vi "Measurement Logic.vi"(8 "error in":errorcluster, 10 "Measurement Context":refnum<class "MeasurementContext.lvclass">, 11 "Measurement Configuration":T2={"delay"=10.0}) -> (0 "error out":errorcluster, 2 "Measurement Context out":refnum<class "MeasurementContext.lvclass">, 3 "Measurement Results":T1)   [LabVIEW 2020, in "CancellableMeasurementProxy.lvlib"]
uses:
  CancellableMeasurementProxy.lvlib
  Measurement Configuration.ctl
  Measurement Results.ctl
  RPC Service/MeasurementContext/MeasurementContext.lvclass
  <vilib>/MeasurementLink/Discovery Client/RPC Messages/ni_measurementlink_discovery_v1_ResolveServiceRequest.ctl
  Measurement Client_lv/Measurement_client/RPC Messages/ni_measurementlink_measurement_v1_MeasureRequest.ctl
  Measurement Client_lv/Measurement_client/RPC Messages/google_protobuf_Any.ctl
  Measurement Client_lv/Measurement_client/RPC Messages/ni_measurementlink_PinMapContext.ctl
  5cd0f8b4-e5f8-4204-8add-725bbbd3d453.vi
  d93fa0da-b198-4c2c-a1c3-c340aeb95d8d.vi
  <vilib>/gRPC/LabVIEW gRPC Library/Server API/Translate Protobuf Error.vi
  <vilib>/AdvancedString/1D String Array to Delimited String.vi
  <vilib>/gRPC/LabVIEW gRPC Library/Server API/Server/Get Server DLL Path.vi
  RPC Service/MeasurementContext/Accessor/Is Canceled.vi
  <vilib>/MeasurementLink/Discovery Client/Discovery_client.lvlib
  Measurement Client_lv/Measurement_client/Measurement_client.lvlib
  <vilib>/gRPC/LabVIEW gRPC Library/grpc-lvsupport-release.lvlib
panel:
  out "target address":string
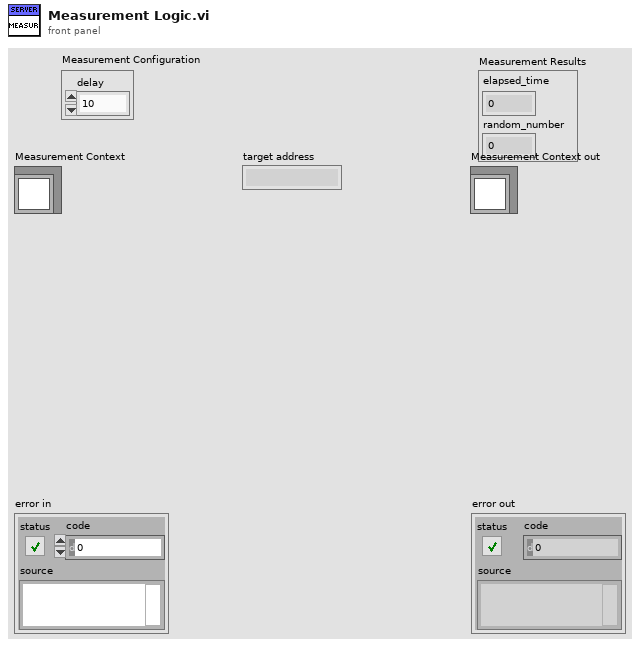
[diagram p1: front panel]
types:
  T1 = typedef "CancellableMeasurementProxy.lvlib/Measurement Results.ctl" = cluster{"elapsed_time":dbl, "random_number":dbl}
  T2 = typedef "CancellableMeasurementProxy.lvlib/Measurement Configuration.ctl" = cluster{"delay":dbl}
  T3 = typedef "Measurement_client.lvlib/ni_measurementlink_measurement_v1_MeasureRequest.ctl" = cluster{"configuration_parameters":T4, "pin_map_context":T5}
  T4 = typedef "Measurement_client.lvlib/google_protobuf_Any.ctl" = cluster{"type_url":string, "value":u8[]}
  T5 = typedef "Measurement_client.lvlib/ni_measurementlink_PinMapContext.ctl" = cluster{"pin_map_id":string, "sites":i32[]}
  T6 = typedef "Discovery_client.lvlib/ni_measurementlink_discovery_v1_ResolveServiceRequest.ctl" = cluster{"provided_interface":string, "service_class":string}
  T7 = typedef "grpc-lvsupport-release.lvlib/grpcId.ctl" = u64
  T8 = typedef "Discovery_client.lvlib/ni_measurementlink_discovery_v1_ServiceLocation.ctl" = cluster{"location":string, "insecure_port":string, "ssl_authenticated_port":string}
  T9 = typedef "grpc-lvsupport-release.lvlib/Any.ctl" = cluster{"Type Url":string, "Bytes":u8[]}
  T10 = typedef "Measurement_client.lvlib/ni_measurementlink_measurement_v1_MeasureResponse.ctl" = cluster{"outputs":T4}
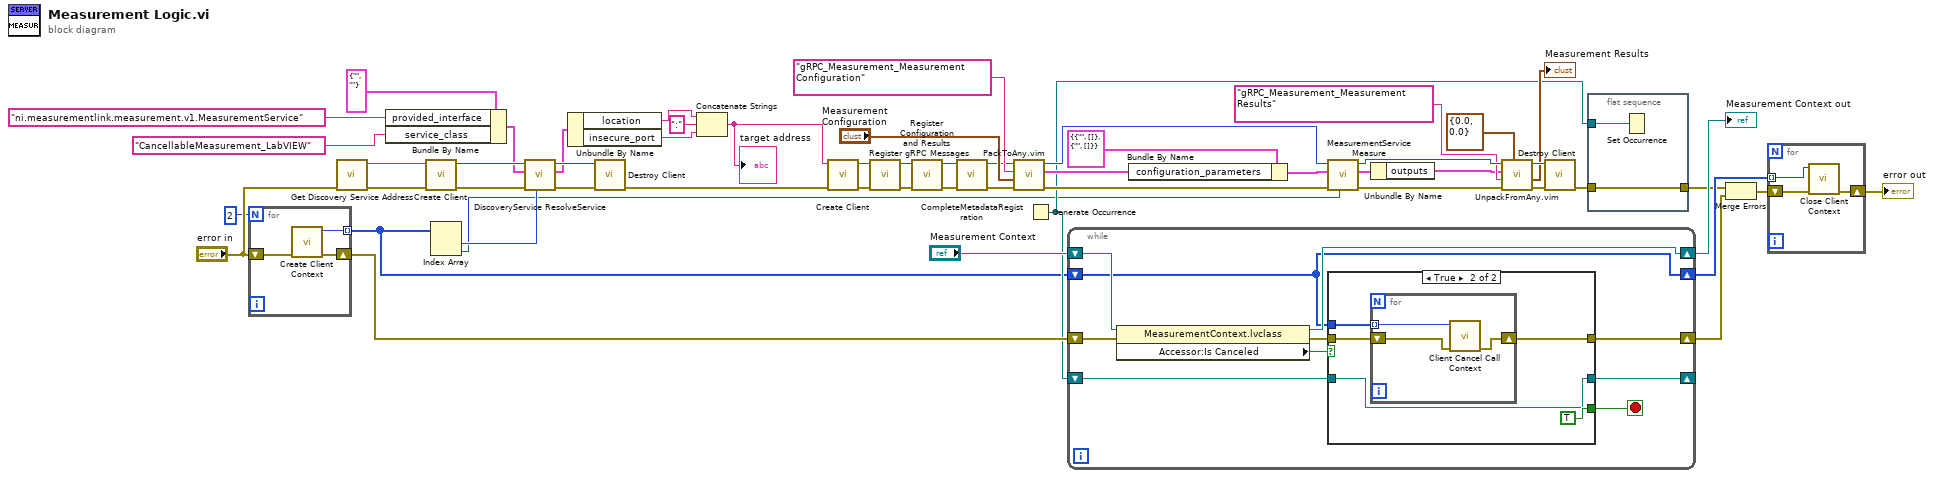
[diagram p0: block diagram]
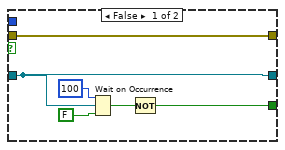
[diagram p2: hidden frame]
diagram:
  n1 = for {
    N: 2 -> [_]
    tunnel: [w57] -> w2 mode=indexing
    shift-right: [w56] -> w14
    shift-left: "error in" -> [w58]
    n2 = call <vilib>:"Create Client Context.vi"("error in (no error)"=w58) -> ("error out"=w56:errorcluster, "ContextID out"=w57:T7)  [unwired: 9 in]
  }
  n3 = call "Get Discovery Service Address.vi"("error in"="error in") -> ("error out"=w46:errorcluster, "address"=w55:string)  [unwired: 9 in]
  n4 = Bundle By Name(cluster=T6 {"provided_interface"="", "service_class"=""} ("Request Data"), "provided_interface"="ni.measurementlink.measurement.v1.MeasurementService", "service_class"="CancellableMeasurement_LabVIEW") -> (w52:T6)
  n5 = call <vilib>:"Create Client.vi"("error in"=w46, "address"=w55) -> ("error out"=w47:errorcluster, "gRPC ID Out"=w54:T7)  [unwired: 8 in]
  n6 = Index Array(array=w2) -> (element #1=w4:T7, element #2=w3:T7)  [unwired: 2 in]
  n7 = call <vilib>:"DiscoveryService ResolveService.vi"("contextId"=w4, "error in"=w47, "Request Data"=w52, "gRPC ID"=w54) -> ("error out"=w48:errorcluster, "Response Data"=w45:T8, "gRPC ID out"=w49:T7)  [unwired: 5 in]
  n8 = Unbundle By Name(w45) -> ("location"=w43:string, "insecure_port"=w42:string)
  n9 = call <vilib>:"Destroy Client.vi"("error in"=w48, "gRPC ID"=w49) -> ("error out"=w16:errorcluster)  [unwired: 9 in]
  n10 = Concatenate Strings(w43, ":" ("string"), w42) -> (w17:string)
  "target address" <- w17
  n11 = call <vilib>:"Create Client.vi"("error in"=w16, "address"=w17) -> ("error out"=w25:errorcluster, "ClientID out"=w24:T7)  [unwired: 8 in]
  n12 = call "Register gRPC Messages.vi"("error in (no error)"=w25, "gRPC ID"=w24) -> ("error out"=w22:errorcluster, "gRPC ID Out"=w23:T7)  [unwired: 8 in]
  n13 = call "Register Configuration and Results.vi"("error in (no error)"=w22, "gRPC ID"=w23) -> ("error out"=w21:errorcluster, "gRPC ID Out"=w20:T7)  [unwired: 8 in]
  n14 = call <vilib>:"CompleteMetadataRegistration.vi"("error in"=w21, "gRPC ID in"=w20) -> ("error out"=w18:errorcluster, "gRPC ID Out"=w19:T7)  [unwired: 8 in]
  n15 = call "PackToAny.vim"("error in"=w18, "Data To Pack"="Measurement Configuration", "Message Type"="gRPC_Measurement_Measurement Configuration", "gRPCid in"=w19) -> ("error out"=w28:errorcluster, "Any"=w36:T9, "gRPCid out"=w41:u64)  [unwired: 5 in]
  n16 = Generate Occurrence() -> (w9:refnum<k4>)
  n17 = while {
    shift-right: [w61] -> w13
    shift-left: w2 -> [w61]
    shift-right: [w65] -> w11
    shift-left: "Measurement Context" -> [w68]
    shift-right: [w63] -> w7
    shift-left: w14 -> [w66]
    shift-right: [w59] -> _
    shift-left: w9 -> [w60]
    stop <- w62 stop-if-true
    n18 = property class="MeasurementContext.lvclass"(reference=w68, error in=w66) -> (reference out=w65:refnum<class "MeasurementContext.lvclass">, error out=w64:errorcluster, "Accessor:Is Canceled"=w67:bool)
    n19 = case shown="True" w67 {
      tunnel: w61 -> [_ w79]
      tunnel: w64 -> [w74 w78]
      tunnel: [w74 w77] -> w63
      tunnel: [w71 TRUE] -> w62
      tunnel: w60 -> [w70 w75]
      tunnel: [w70 w75] -> w59
      frame False {
        n20 = Wait on Occurrence(1:FALSE ("ignore previous (T)"), 2:w70, 3:100 ("ms timeout (-1)")) -> (0:w72:bool)
        n21 = Not(x=w72) -> (.not. x?=w71:bool)
      }
      frame True {
        n22 = for {
          tunnel: w79 -> [w82] mode=indexing
          shift-right: [w80] -> w77
          shift-left: w78 -> [w81]
          n23 = call <vilib>:"Client Cancel Call Context.vi"("error in"=w81, "Call ID in"=w82) -> ("error out"=w80:errorcluster)  [unwired: 9 in]
        }
      }
    }
  }
  "Measurement Context out" <- w11
  n24 = Bundle By Name(cluster=T3 {"configuration_parameters"={"type_url"="", "value"=[]}, "pin_map_context"={"pin_map_id"="", "sites"=[]}} ("Request Data"), "configuration_parameters"=w36) -> (w37:T3)
  n25 = call "MeasurementService Measure.vi"("contextId"=w3, "error in"=w28, "Request Data"=w37, "gRPC ID"=w41) -> ("error out"=w27:errorcluster, "Response Data"=w33:T10, "gRPC ID out"=w35:T7)  [unwired: 5 in]
  n26 = Unbundle By Name(w33) -> ("outputs"=w32:T4)
  n27 = call "UnpackFromAny.vim"("Data Type"=T1 {"elapsed_time"=0.0, "random_number"=0.0} ("Measurement Results"), "error in"=w27, "Message Type"="gRPC_Measurement_Measurement Results", "Any"=w32, "gRPCid in"=w35) -> ("error out"=w26:errorcluster, "Unpacked Value"=→"Measurement Results":T1, "gRPCid out"=w31:u64)  [unwired: 4 in]
  n28 = call <vilib>:"Destroy Client.vi"("error in"=w26, "gRPC ID"=w31) -> ("error out"=w10:errorcluster)  [unwired: 9 in]
  n29 = flat-sequence {
    tunnel: [w84] -> w8
    tunnel: w10 -> [w84]
    tunnel: w9 -> [w83]
    frame #0 {
      n30 = Set Occurrence(w83) -> ()
    }
  }
  n31 = Merge Errors(w8, w7) -> (w6:errorcluster)
  n32 = for {
    tunnel: w13 -> [w87] mode=indexing
    shift-right: [w85] -> w5
    shift-left: w6 -> [w86]
    n33 = call <vilib>:"Close Client Context.vi"("error in (no error)"=w86, "ContextID"=w87) -> ("error out"=w85:errorcluster)  [unwired: 9 in]
  }
  "error out" <- w5
